vi "save_data_start.vi"(5 "Save Video":bool, 6 "Frames Per Second":u32) -> (1 "Saving":bool, 2 "Avi Refnum":T1, 3 "Data Refnum":refnum<file>)   [LabVIEW 2019]
doc: "This VI opens files to which we can save data and, optionally, video. It handles auto-incrementing numbers in filenames (if present) and should handle errors nicely."
uses:
  <vilib>/vision/Avi1.llb/AviRefnum.ctl
  <vilib>/regexp/Match Regular Expression.xnode
panel:
  in  "start path":path=path ""
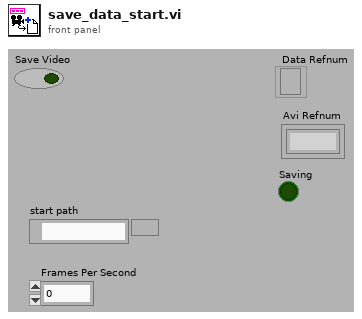
[diagram p1: front panel]
types:
  T1 = typedef "AviRefnum.ctl" = refnum<k1>
  T2 = enum16{"open", "replace", "create", "open or create", "replace or create", "replace or create with confirmation"}
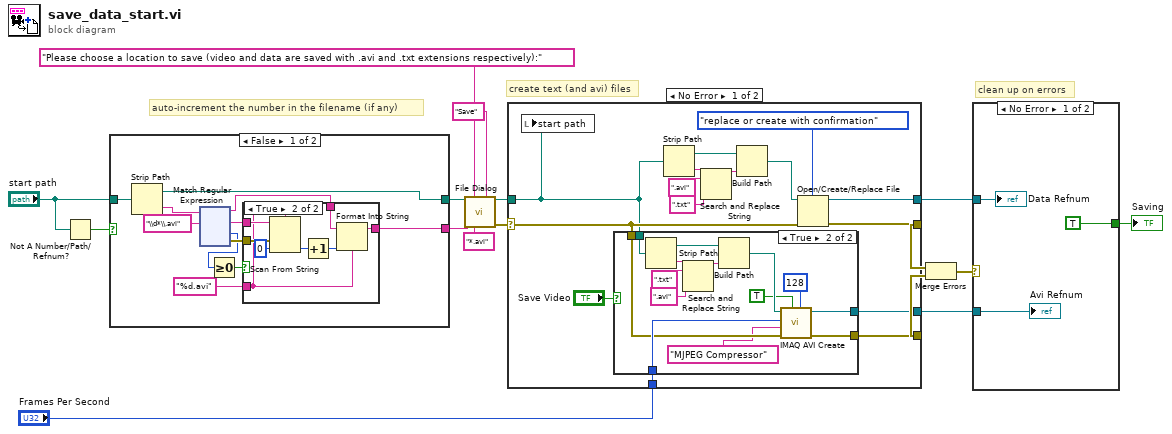
[diagram p0: block diagram]
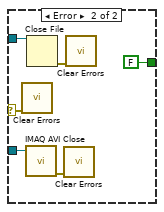
[diagram p2: hidden frame]
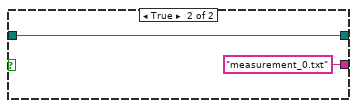
[diagram p6: hidden frame]
diagram:
  # "clean up on errors"
  # "create text (and avi) files"
  # "auto-increment the number in the filename (if any)"
  n1 = Not A Number/Path/Refnum?(number/path/refnum="start path") -> (NaN/Path/Refnum?=w12:bool)
  n2 = case shown="False" w12 {
    tunnel: "start path" -> [w27 w149]
    tunnel: [w17 w149] -> w13
    tunnel: [w18 "measurement_0.txt" ("before match")] -> w15
    frame False {
      n3 = Strip Path(path=w27) -> (stripped path=w17:path, name=w26:string)
      n4 = xnode "Match Regular Expression"("input string"=w26, "regular expression"="\\d*\\.avi") -> ("before match"=w21:string, "whole match"=w23:string, "offset past match"=w19:i32, "error out"=w24:errorcluster)  [unwired: 4 in, 1 out]
      n5 = Greater Or Equal To 0?(x=w19) -> (x >= 0?=w20:bool)
      n6 = case shown="True" w20 {
        tunnel: w24 -> [_ w36]
        tunnel: w23 -> [_ w35]
        tunnel: "%d.avi" ("format string") -> [_ w30]
        tunnel: w21 -> [w28 w31]
        tunnel: [w28 w29] -> w18
        frame False {
        }
        frame True {
          n7 = Scan From String(format string=w30, input string=w35, error in=w36, default 1=0 ("default value 1")) -> (output 1=w34:i32)  [unwired: 1 in, 3 out]
          n8 = Increment(x=w34) -> (x+1=w32:i32)
          n9 = Format Into String(format string=w30, initial string=w31, w32) -> (resulting string=w29:string)  [unwired: 1 in, 1 out]
        }
      }
    }
    frame True {
    }
  }
  n10 = call "File Dialog"("start path"=w13, "prompt"="Please choose a location to save (video and data are saved with .avi and .txt extensions respectively):", "button label"="Save", "default name"=w15, "pattern (all files)"="*.avi") -> ("selected path"=w10:path, "error out"=w9:errorcluster)  [unwired: 7 in, 2 out]
  n11 = case shown="No Error" w9 {
    selector: w9 -> [w163 w179]
    tunnel: "Frames Per Second" -> [w164 _]
    tunnel: w10 -> [w151 _]
    tunnel: [w161 w179] -> w7
    tunnel: [w160 w179] -> w5
    tunnel: [w159 _] -> w4
    tunnel: [w158 _] -> w3
    frame No Error {
      n12 = local write "start path"(w151) -> ()
      n13 = case shown="True" "Save Video" {
        tunnel: w164 -> [_ w178]
        tunnel: w163 -> [_ w177]
        tunnel: w151 -> [_ w176]
        tunnel: [_ w167] -> w160
        tunnel: [_ w166] -> w159
        frame False {
        }
        frame True {
          n14 = Strip Path(path=w176) -> (stripped path=w171:path, name=w175:string)
          n15 = Search and Replace String(input string=w175, search string=".txt", replace string=".avi" ("replace string (\"\")")) -> (result string=w172:string)  [unwired: 5 in, 3 out]
          n16 = Build Path(base path=w171, name or relative path=w172) -> (appended path=w170:path)
          n17 = call "IMAQ AVI Create"("Max Data Size"=u32 128, "Has Data"=TRUE, "error in (no error)"=w177, "Compression Filter"="MJPEG Compressor", "Frames Per Second"=w178, "AVI Path"=w170) -> ("error out"=w167:errorcluster, "Avi Refnum"=w166:T1)  [unwired: 4 in]
        }
      }
      n18 = Strip Path(path=w151) -> (stripped path=w152:path, name=w156:string)
      n19 = Search and Replace String(input string=w156, search string=".avi", replace string=".txt" ("replace string (\"\")")) -> (result string=w153:string)  [unwired: 5 in, 3 out]
      n20 = Build Path(base path=w152, name or relative path=w153) -> (appended path=w150:path)
      n21 = Open/Create/Replace File(file path (use dialog)=w150, error in=w163, operation (0:open)=T2."replace or create with confirmation") -> (refnum out=w158:refnum<file>, error out=w161:errorcluster)  [unwired: 3 in, 1 out]
    }
    frame Error {
    }
  }
  n22 = Merge Errors(w7, w5) -> (w6:errorcluster)
  n23 = case shown="No Error" w6 {
    selector: w6 -> [_ w187]
    tunnel: [TRUE FALSE] -> w8
    tunnel: w4 -> [w181 w184]
    tunnel: w3 -> [w180 w186]
    frame No Error {
      "Avi Refnum" <- w181
      "Data Refnum" <- w180
    }
    frame Error {
      n24 = call <vilib>:"Clear Errors.vi"("error in (no error)"=w187) -> ()  [unwired: 5 in, 2 out]
      n25 = call "IMAQ AVI Close"("Avi Refnum"=w184) -> ("error out"=w183:errorcluster)  [unwired: 10 in]
      n26 = Close File(refnum=w186) -> (error out=w185:errorcluster)  [unwired: 1 in, 1 out]
      n27 = call <vilib>:"Clear Errors.vi"("error in (no error)"=w183) -> ()  [unwired: 5 in, 2 out]
      n28 = call <vilib>:"Clear Errors.vi"("error in (no error)"=w185) -> ()  [unwired: 5 in, 2 out]
    }
  }
  "Saving" <- w8
